vi "Initialize DAQ Events.vi"(8 "error in (no error)":errorcluster, 11 "DAQ":refnum<class "DAQ.lvclass">) -> (0 "error out":errorcluster, 3 "DAQ":refnum<class "DAQ.lvclass">)   [LabVIEW 2022 SP3, in "DAQ.lvclass"]
doc: "Developed by Kevin Thompson\nkevin@thompsonengineering.net\n\nCopyright 2018-2020\nThompson Engineering, LLC"
uses:
  DAQ.lvclass
  Process/ProcessSupport/TD DAQ Output Cmd EventData--cluster.ctl
  Process/ProcessSupport/TD DaqOutCmd--enum.ctl
  DataTypes/TD DAQ Output EventSenderMode-enum.ctl
  Common/Controls/TD Async CmdMsg EventData--cluster.ctl
  DataTypes/TD DAQStateChanged EventData--cluster.ctl
  DataTypes/TD DAQ&TDMS State Data--cluster.ctl
  DataTypes/TD DaqState--enum.ctl
  DAQ.lvclass/DAQ.ctl
  DataTypes/TD DAQ DI state change ev.ctl
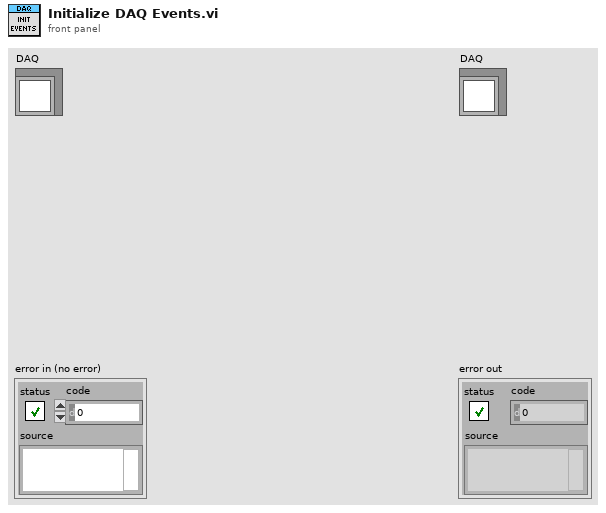
[diagram p1: front panel]
types:
  T1 = typedef "DAQ.lvclass/TD DAQStateChanged EventData--cluster.ctl" = cluster{"Time Stamp":timestamp, "OLD State Data":T2, "NEW State Data":T2}
  T2 = typedef "DAQ.lvclass/TD DAQ&TDMS State Data--cluster.ctl" = cluster{"DAQState":T3, "vData":variant}
  T3 = typedef "DAQ.lvclass/TD DaqState--enum.ctl" = enum16{"Unknown", "Stopped", "Running", "Error"}
  T4 = typedef "TD DAQ DI state change ev.ctl" = cluster{"Time Stamp":timestamp, "Name":string, "vData":variant}
  T5 = typedef "TD Async CmdMsg EventData--cluster.ctl" = cluster{"Time Stamp":timestamp, "CmdMsg":string, "vData":variant}
  T6 = typedef "DAQ.lvclass/TD DAQ Output Cmd EventData--cluster.ctl" = cluster{"TimeStamp":dbl, "DaqOutCmd":T7, "IOName":string, "BoolState":bool, "AnalogVal":dbl, "WaitTime (ms)":u32, "mode":T8, "vData":variant}
  T7 = typedef "DAQ.lvclass/TD DaqOutCmd--enum.ctl" = enum16{"Set DO", "Set AO", "Toggle DO", "Invert DO"}
  T8 = typedef "DAQ.lvclass/TD DAQ Output EventSenderMode-enum.ctl" = enum16{"manual", "automation"}
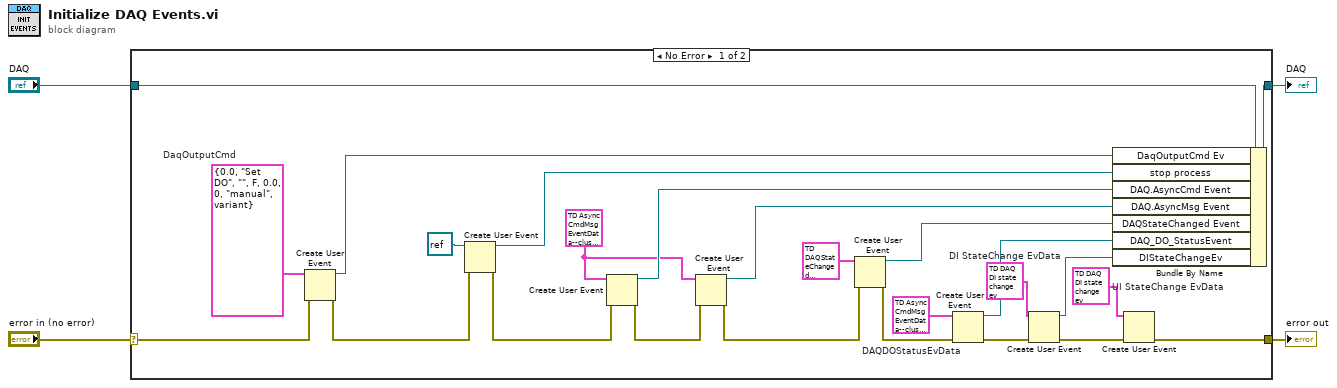
[diagram p0: block diagram]
diagram:
  n1 = case shown="No Error" "error in (no error)" {
    selector: "error in (no error)" -> [w27 w31]
    tunnel: [w5 w31] -> w3
    tunnel: [w28 w30] -> w1
    tunnel: "DAQ" -> [w29 w30]
    frame No Error {
      w7 = T4 {"Time Stamp"=timestamp(0 s since 1904-01-01), "Name"="", "vData"=variant}  # UI StateChange EvData
      w10 = T4 {"Time Stamp"=timestamp(0 s since 1904-01-01), "Name"="", "vData"=variant}  # DI StateChange EvData
      w13 = T5 {"Time Stamp"=timestamp(0 s since 1904-01-01), "CmdMsg"="", "vData"=variant}  # DAQDOStatusEvData
      w17 = T5 {"Time Stamp"=timestamp(0 s since 1904-01-01), "CmdMsg"="", "vData"=variant} ("Async EvData")
      w26 = T6 {"TimeStamp"=0.0, "DaqOutCmd"=enum."Set DO", "IOName"="", "BoolState"=FALSE, "AnalogVal"=0.0, "WaitTime (ms)"=0, "mode"=enum."manual", "vData"=variant}  # DaqOutputCmd
      n2 = Create User Event(user event datatype=w26, error in=w27) -> (user event=w25:refnum<user-event>, error out=w22:errorcluster)
      n3 = Create User Event(user event datatype=refnum<notifier> refnum ("notifier out"), error in=w22) -> (user event=w23:refnum<user-event>, error out=w21:errorcluster)
      n4 = Create User Event(user event datatype=w17, error in=w21) -> (user event=w20:refnum<user-event>, error out=w15:errorcluster)
      n5 = Create User Event(user event datatype=w17, error in=w15) -> (user event=w16:refnum<user-event>, error out=w14:errorcluster)
      n6 = Create User Event(user event datatype=T1 {"Time Stamp"=timestamp(0 s since 1904-01-01), "OLD State Data"={"DAQState"=enum."Stopped", "vData"=variant}, "NEW State Data"={"DAQState"=enum."Stopped", "vData"=variant}} ("DAQStateChanged EventData"), error in=w14) -> (user event=w18:refnum<user-event>, error out=w12:errorcluster)
      n7 = Create User Event(user event datatype=w13, error in=w12) -> (user event=w11:refnum<user-event>, error out=w9:errorcluster)
      n8 = Create User Event(user event datatype=w10, error in=w9) -> (user event=w8:refnum<user-event>, error out=w6:errorcluster)
      n9 = Bundle By Name(cluster=w29, "DaqOutputCmd Ev"=w25, "stop process"=w23, "DAQ.AsyncCmd Event"=w20, "DAQ.AsyncMsg Event"=w16, "DAQStateChanged Event"=w18, "DAQ_DO_StatusEvent"=w11, "DIStateChangeEv"=w8) -> (w28:refnum<class "DAQ.lvclass">)
      n10 = Create User Event(user event datatype=w7, error in=w6) -> (error out=w5:errorcluster)  [unwired: 1 out]
    }
    frame Error {
    }
  }
  "error out" <- w3
  "DAQ" <- w1
